vi "DN4_1DarrayTo2Darray.vi"(2 "row count":i32, 3 "1Darray":dbl[](array[numeric])) -> (1 "2Darray":dbl[][](array[numeric]))   [LabVIEW 2009]
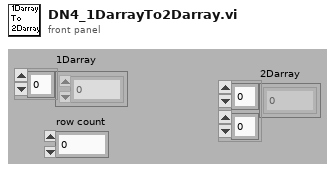
[diagram p1: front panel]
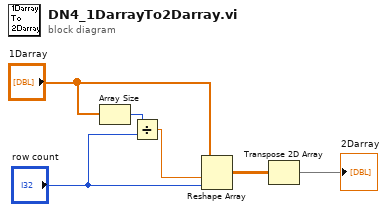
[diagram p0: block diagram]
diagram:
  n1 = Array Size(array="1Darray") -> (size(s)=w3:i32)
  n2 = Divide(x=w3, y="row count") -> (x/y=w2:dbl)
  n3 = Reshape Array("1Darray", w2, "row count") -> (w1:dbl[][])
  n4 = Transpose 2D Array(2D array=w1) -> (transposed array=→"2Darray":dbl[][])
